vi "Set Scale Label.vi"(8 "error in (no error)":errorcluster, 11 "[V] Waveform in":refnum<class "[V] Waveform.lvclass">) -> (0 "error out":errorcluster, 3 "[V] Waveform out":refnum<class "[V] Waveform.lvclass">)   [LabVIEW 2023, in "[V] Waveform.lvlib" / "[V] Waveform.lvclass"]
uses:
  [V] Waveform.lvclass
  [V] Waveform.lvclass/[V] Waveform.ctl
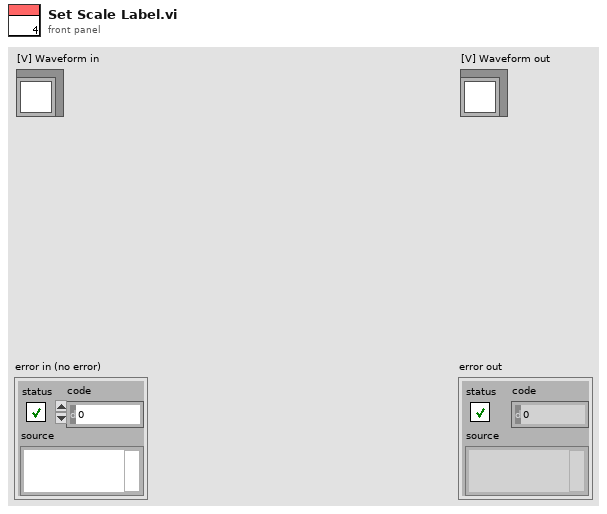
[diagram p1: front panel]
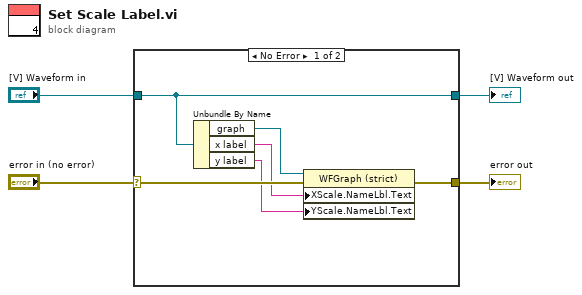
[diagram p0: block diagram]
diagram:
  n1 = case shown="No Error" "error in (no error)" {
    selector: "error in (no error)" -> [w9 w12]
    tunnel: [w7 w12] -> w3
    tunnel: [w10 w11] -> w1
    tunnel: "[V] Waveform in" -> [w10 w11]
    frame No Error {
      n2 = Unbundle By Name(w10) -> ("graph"=w8:refnum<vi>, "x label"=w6:string, "y label"=w5:string)
      n3 = property class="WFGraph (strict)"(reference=w8, error in=w9, "XScale.NameLbl.Text"=w6, "YScale.NameLbl.Text"=w5) -> (error out=w7:errorcluster)  [unwired: 1 out]
    }
    frame Error {
    }
  }
  "error out" <- w3
  "[V] Waveform out" <- w1
